vi "niDTS BT INSTR RX Configure BT Payload.vi"(8 "error in (no error)":errorcluster, 11 "niDTS BT INSTR RX in":refnum<class "niDTS BT INSTR RX.lvclass">) -> (0 "error out":errorcluster, 3 "niDTS BT INSTR RX out":refnum<class "niDTS BT INSTR RX.lvclass">)   [LabVIEW 2015, in "niDTS BT.lvlib" / "niDTS BT INSTR RX.lvclass"]
uses:
  niDTS BT INSTR RX.lvclass
  niDTS BT INSTR RX.lvclass/niDTS BT INSTR RX.ctl
  RiviInstDriver/niRfsgBT/Objects/niRfsgBt.lvclass
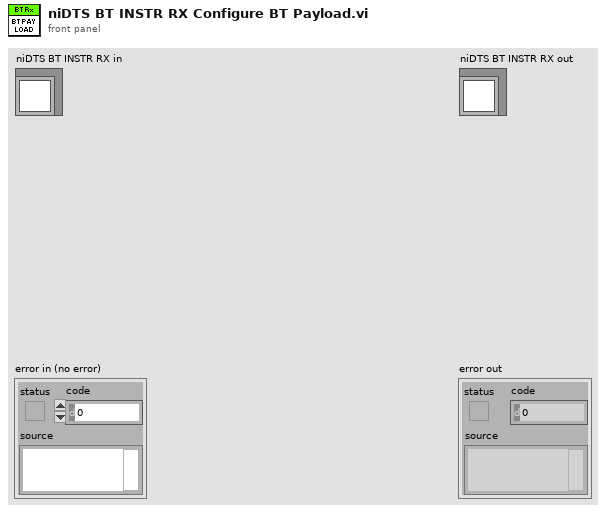
[diagram p1: front panel]
types:
  T1 = typedef "niRfsgBT.lvclass/niRfsgBT INC Handle.ctl" = refnum<data-value>
  T2 = typedef "niDTS BT.lvlib/niDTS BT Tx Test INC BD Payload Data.ctl" = enum16{"0", "1", "01", "00001111", "PN9", "AUTO"}
  T3 = typedef "niDTS BT.lvlib/niDTS BT Rx Test INC Carrier Mode.ctl" = enum16{"Burst", "Continuous"}
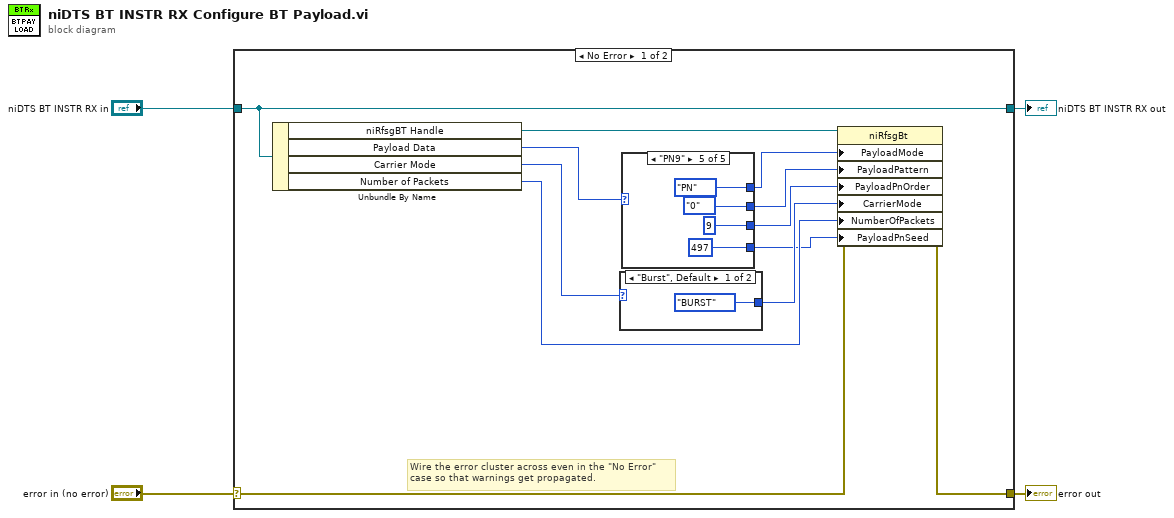
[diagram p0: block diagram]
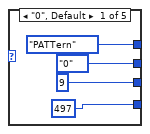
[diagram p2: hidden frame]
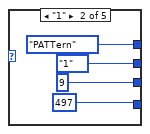
[diagram p3: hidden frame]
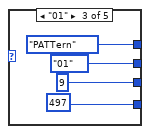
[diagram p4: hidden frame]
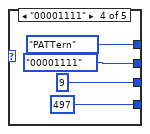
[diagram p5: hidden frame]
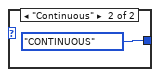
[diagram p6: hidden frame]
diagram:
  n1 = case shown="No Error" "error in (no error)" {
    selector: "error in (no error)" -> [w12 w40]
    tunnel: [w11 w40] -> w3
    tunnel: [w15 w39] -> w1
    tunnel: "niDTS BT INSTR RX in" -> [w15 w39]
    frame No Error {
      # "Wire the error cluster across even in the \"No Error\"\ncase so that warnings get propagated."
      n2 = Unbundle By Name(w15) -> ("niRfsgBT Handle"=w16:T1, "Payload Data"=w13:T2, "Carrier Mode"=w14:T3, "Number of Packets"=w10:i32)
      n3 = case shown="\"Burst\", Default" w14 {
        tunnel: [enum16{"BURST", "CONTINUOUS"}."BURST" ("SOURce:RFSG:BLUetooth:CARRier:CarrierMode") enum16{"BURST", "CONTINUOUS"}."CONTINUOUS" ("SOURce:RFSG:BLUetooth:CARRier:CarrierMode")] -> w6
        frame "Burst", Default {
        }
        frame "Continuous" {
        }
      }
      n4 = case shown="\"PN9\"" w13 {
        tunnel: [enum16{"PN", "PATTern", "USER"}."PATTern" ("SOURce:RFSG:BLUetooth:PACKet:PAYLoad:Mode_A") enum16{"PN", "PATTern", "USER"}."PATTern" ("SOURce:RFSG:BLUetooth:PACKet:PAYLoad:Mode_A") enum16{"PN", "PATTern", "USER"}."PATTern" ("SOURce:RFSG:BLUetooth:PACKet:PAYLoad:Mode_A") enum16{"PN", "PATTern", "USER"}."PATTern" ("SOURce:RFSG:BLUetooth:PACKet:PAYLoad:Mode_A") enum16{"PN", "PATTern", "USER"}."PN" ("SOURce:RFSG:BLUetooth:PACKet:PAYLoad:Mode_A")] -> w9
        tunnel: [enum16{"0", "1", "01", "0011", "00001111"}."0" ("SOURce:RFSG:BLUetooth:PACKet:PAYLoad:PayloadPattern_A") enum16{"0", "1", "01", "0011", "00001111"}."1" ("SOURce:RFSG:BLUetooth:PACKet:PAYLoad:PayloadPattern_A") enum16{"0", "1", "01", "0011", "00001111"}."01" ("SOURce:RFSG:BLUetooth:PACKet:PAYLoad:PayloadPattern_A") enum16{"0", "1", "01", "0011", "00001111"}."00001111" ("SOURce:RFSG:BLUetooth:PACKet:PAYLoad:PayloadPattern_A") enum16{"0", "1", "01", "0011", "00001111"}."0" ("SOURce:RFSG:BLUetooth:PACKet:PAYLoad:PayloadPattern_A")] -> w8
        tunnel: [9 ("SOURce:RFSG:BLUetooth:PACKet:PAYLoad:PN:PnOrder_A") 9 ("SOURce:RFSG:BLUetooth:PACKet:PAYLoad:PN:PnOrder_A") 9 ("SOURce:RFSG:BLUetooth:PACKet:PAYLoad:PN:PnOrder_A") 9 ("SOURce:RFSG:BLUetooth:PACKet:PAYLoad:PN:PnOrder_A") 9 ("SOURce:RFSG:BLUetooth:PACKet:PAYLoad:PN:PnOrder_A")] -> w7
        tunnel: [497 ("SOURce:RFSG:BLUetooth:PACKet:PAYLoad:PN:PnOrder_A") 497 ("SOURce:RFSG:BLUetooth:PACKet:PAYLoad:PN:PnOrder_A") 497 ("SOURce:RFSG:BLUetooth:PACKet:PAYLoad:PN:PnOrder_A") 497 ("SOURce:RFSG:BLUetooth:PACKet:PAYLoad:PN:PnOrder_A") 497 ("SOURce:RFSG:BLUetooth:PACKet:PAYLoad:PN:PnOrder_A")] -> w5
        frame "0", Default {
        }
        frame "1" {
        }
        frame "01" {
        }
        frame "00001111" {
        }
        frame "PN9" {
        }
      }
      n5 = property class="niRfsgBt"(reference=w16, error in=w12, "PayloadMode"=w9, "PayloadPattern"=w8, "PayloadPnOrder"=w7, "CarrierMode"=w6, "NumberOfPackets"=w10, "PayloadPnSeed"=w5) -> (error out=w11:errorcluster)  [unwired: 1 out]
    }
    frame Error {
    }
  }
  "error out" <- w3
  "niDTS BT INSTR RX out" <- w1
